vi "create plot history data.vi"(11 "cluster in":T1={"rigChannels"=[], "rigUnits"=[], "logging"=FALSE, "chartRef"=refnum, "dataTableRef"=refnum, "channelCount"=0, "trendIndex"=0, "channels"={"massflow"=0, "PR"=0, "recircTemp"=0}, "History"={"speedlines"=[], "liveTail"={"mDot"=[], "pRatio"=[]}, "current"={"mDot"=0.0, "pRatio"=0.0}, "insertPoint"=0, "tempHistory"=[]}, "filter"=FALSE, "filterLength"=0, "tableUpdate"=0, "limitValues"=[[0.0, 45000.0], [0.0, 100.0], [0.0, 100.0], [10.0, 100.0], [0.0, 100.0], [10.0, 35.0], [0.0, 100.0], [0.0, 100.0], [99000.0, 300000.0], [-5000.0, 5000.0], [99000.0, 300000.0], [-0.01, 0.3], [-0.01, 4.5], [-0.1, 100.0], [1.0, 8.0], [1.0, 5.0], [0.0, 100.0], [0.0, 100.0], [0.0, 100.0], [-100.0, 45000.0], [-0.1, 1.0], [0.8, 2.0], [90000.0, 110000.0], [15.0, 35.0], [0.0, 0.0], [0.0, 0.0], [0.0, 0.0], [0.0, 0.0]]}) -> (2 "cluster out 2":T1={"rigChannels"=[], "rigUnits"=[], "logging"=FALSE, "chartRef"=refnum, "dataTableRef"=refnum, "channelCount"=0, "trendIndex"=0, "channels"={"massflow"=0, "PR"=0, "recircTemp"=0}, "History"={"speedlines"=[], "liveTail"={"mDot"=[], "pRatio"=[]}, "current"={"mDot"=0.0, "pRatio"=0.0}, "insertPoint"=0, "tempHistory"=[]}, "filter"=FALSE, "filterLength"=0, "tableUpdate"=0, "limitValues"=[[0.0, 45000.0], [0.0, 100.0], [0.0, 100.0], [10.0, 100.0], [0.0, 100.0], [10.0, 35.0], [0.0, 100.0], [0.0, 100.0], [99000.0, 300000.0], [-5000.0, 5000.0], [99000.0, 300000.0], [-0.01, 0.3], [-0.01, 4.5], [-0.1, 100.0], [1.0, 8.0], [1.0, 5.0], [0.0, 100.0], [0.0, 100.0], [0.0, 100.0], [-100.0, 45000.0], [-0.1, 1.0], [0.8, 2.0], [90000.0, 110000.0], [15.0, 35.0], [0.0, 0.0], [0.0, 0.0], [0.0, 0.0], [0.0, 0.0]]}, 3 "Array":cluster{"mDot":dbl[], "pRatio":dbl[]}[](array[cluster]))   [LabVIEW 2018]
uses:
  custom sub vis/speedlineData.ctl
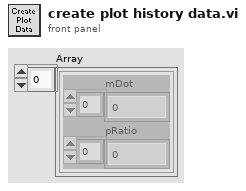
[diagram p1: front panel]
types:
  T1 = typedef "speedlineData.ctl" = cluster{"rigChannels":string[], "rigUnits":string[], "logging":bool, "chartRef":refnum<vi>, "dataTableRef":refnum<vi>, "channelCount":i32, "trendIndex":i32, "channels":cluster{"massflow":i32, "PR":i32, "recircTemp":i32}, "History":cluster{"speedlines":cluster{"mDot":dbl[], "pRatio":dbl[]}[], "liveTail":cluster{"mDot":dbl[], "pRatio":dbl[]}, "current":cluster{"mDot":dbl, "pRatio":dbl}, "insertPoint":i32, "tempHistory":dbl[][]}, "filter":bool, "filterLength":i32, "tableUpdate":i16, "limitValues":dbl[][]}
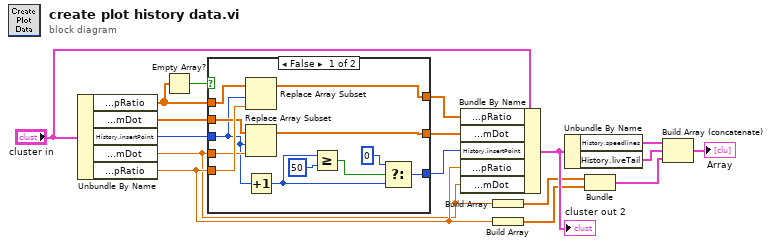
[diagram p0: block diagram]
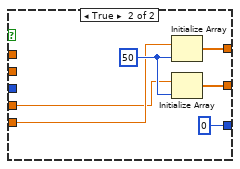
[diagram p2: hidden frame]
diagram:
  n1 = Unbundle By Name("cluster in") -> ("History.liveTail.pRatio"=w6:dbl[], "History.liveTail.mDot"=w7:dbl[], "History.insertPoint"=w10:i32, "History.current.mDot"=w15:dbl, "History.current.pRatio"=w16:dbl)
  n2 = Empty Array?(array=w6) -> (empty?=w5:bool)
  n3 = case shown="False" w5 {
    tunnel: w6 -> [w29 _]
    tunnel: w7 -> [w26 _]
    tunnel: w16 -> [w28 w34]
    tunnel: w15 -> [w25 w33]
    tunnel: [w27 w32] -> w8
    tunnel: [w24 w31] -> w9
    tunnel: w10 -> [w23 _]
    tunnel: [w21 0] -> w11
    frame False {
      n4 = Replace Array Subset(array=w29, new element=w28, index=w23) -> (w27:dbl[])
      n5 = Replace Array Subset(array=w26, new element=w25, index=w23) -> (w24:dbl[])
      n6 = Increment(x=w23) -> (x+1=w19:i32)
      n7 = Greater Or Equal?(x=w19, y=50 ("x")) -> (x >= y?=w22:bool)
      n8 = Select(t=0, s=w22, f=w19) -> (s? t:f=w21:i32)
    }
    frame True {
      w35 = 50 ("dimension size")
      n9 = Initialize Array(w34, w35) -> (w32:dbl[])
      n10 = Initialize Array(w33, w35) -> (w31:dbl[])
    }
  }
  n11 = Bundle By Name(cluster="cluster in", "History.liveTail.pRatio"=w8, "History.liveTail.mDot"=w9, "History.insertPoint"=w11, "History.current.pRatio"=w16, "History.current.mDot"=w15) -> (w14:T1)
  "cluster out 2" <- w14
  n12 = Build Array(w15) -> (w12:dbl[])
  n13 = Build Array(w16) -> (w13:dbl[])
  n14 = Unbundle By Name(w14) -> ("History.speedlines"=w2:cluster{"mDot":dbl[], "pRatio":dbl[]}[], "History.liveTail"=w3:cluster{"mDot":dbl[], "pRatio":dbl[]})
  n15 = Bundle(w12, w13) -> (w4:cluster{dbl[], dbl[]})  [unwired: 1 in]
  n16 = Build Array (concatenate)(w2, w3, w4) -> (→"Array":cluster{"mDot":dbl[], "pRatio":dbl[]}[])
